vi "[Your Turn] Running Average Using Stacked Shift Register.vi"() -> ()   [LabVIEW 2019]
uses:
  <vilib>/DAQmx/read.llb/DAQmx Read (Analog DBL 1Chan 1Samp).vi
  <vilib>/DAQmx/create/channels.llb/DAQmx Create Channel (AI-Temperature-Thermocouple).vi
  <vilib>/DAQmx/configure/timing.llb/DAQmx Timing (Sample Clock).vi
  <vilib>/DAQmx/miscellaneous.llb/DAQmx Fill In Error Info.vi
panel:
  out "Temperature Chart":dbl(graph)
  out "Average Temperature Chart":dbl(graph)
  in  "Stop":bool
  in  "Thermocouple Channel":tag="PCI-6221/ai0"
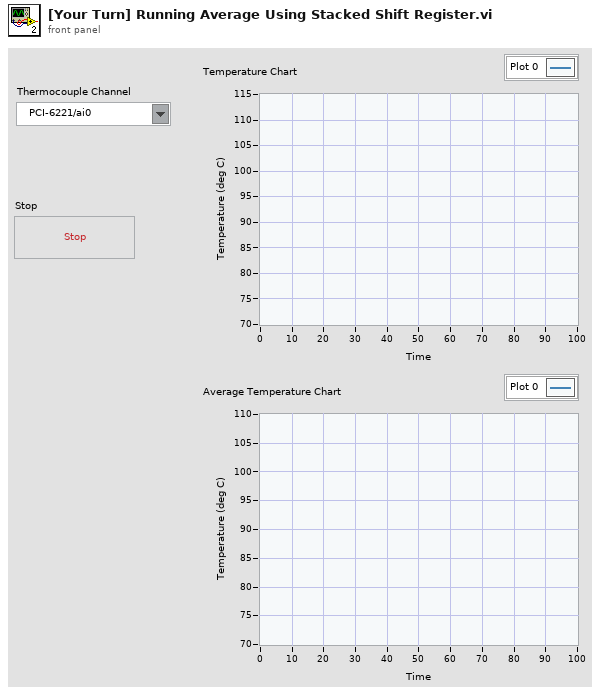
[diagram p1: front panel]
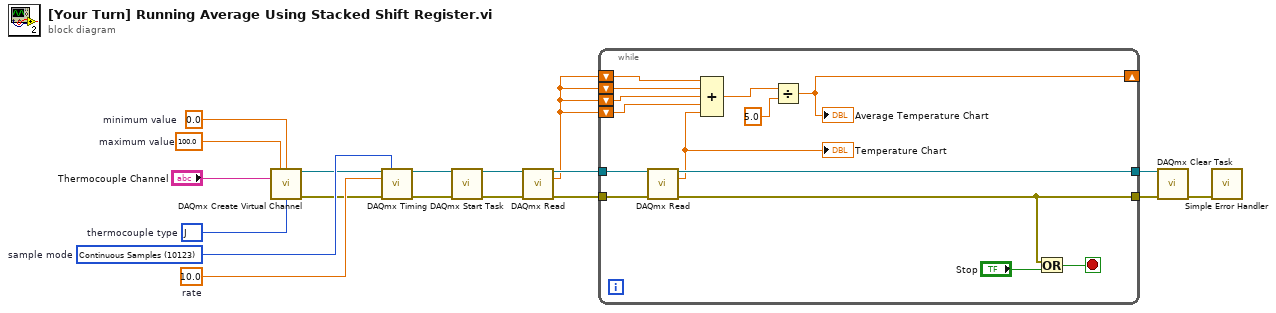
[diagram p0: block diagram]
diagram:
  w7 = 10072 items=["J"=10072, "K"=10073, "N"=10077, "R"=10082, "S"=10085, "T"=10086, "B"=10047, "E"=10055]  # thermocouple type
  w8 = 100.0  # maximum value
  w9 = 0.0  # minimum value
  w17 = 10.0  # rate
  w18 = 10123 items=["Finite Samples"=10178, "Continuous Samples"=10123, "Hardware Timed Single Point"=12522]  # sample mode
  n1 = call-poly <vilib>:"DAQmx Create Virtual Channel.vi"("maximum value"=w8, "minimum value"=w9, "physical channels"="Thermocouple Channel", "thermocouple type"=w7) -> ("task out"=w16:refnum<k21>, "error out"=w15:errorcluster)  [unwired: 10 in]
  n2 = call-poly <vilib>:"DAQmx Timing.vi"("task/channels in"=w16, "sample mode"=w18, "rate"=w17, "error in"=w15) -> ("task out"=w14:refnum<k21>, "error out"=w13:errorcluster)  [unwired: 10 in]
  n3 = call <vilib>:"DAQmx Start Task.vi"("task/channels in"=w14, "error in"=w13) -> ("task out"=w12:refnum<k21>, "error out"=w11:errorcluster)  [unwired: 12 in]
  n4 = call-poly <vilib>:"DAQmx Read.vi"("task/channels in"=w12, "error in"=w11) -> ("task out"=w6:refnum<k21>, "data"=w1:dbl, "error out"=w5:errorcluster)  [unwired: 11 in]
  n5 = while {
    tunnel: w6 -> [w32]
    tunnel: w5 -> [w31]
    shift-right: [w25] -> _
    shift-left: w1 -> [w30]
    shift-left: w1 -> [w29]
    tunnel: [w28] -> w4
    tunnel: [w24] -> w3
    shift-left: w1 -> [w21]
    shift-left: w1 -> [w20]
    stop <- w22 stop-if-true
    n6 = call-poly <vilib>:"DAQmx Read.vi"("task/channels in"=w32, "error in"=w31) -> ("task out"=w28:refnum<k21>, "data"=w19:dbl, "error out"=w24:errorcluster)  [unwired: 11 in]
    "Temperature Chart" <- w19
    n7 = Compound Arithmetic op=ADD(w30, w29, w21, w20, w19) -> (w27:dbl)
    n8 = Divide(x=w27, y=5.0) -> (x/y=w25:dbl)
    "Average Temperature Chart" <- w25
    n9 = Or(x=w24, y="Stop") -> (x .or. y?=w22:bool)
  }
  n10 = call <vilib>:"DAQmx Clear Task.vi"("task in"=w4, "error in"=w3) -> ("error out"=w2:errorcluster)  [unwired: 13 in]
  n11 = call <vilib>:"Simple Error Handler.vi"("error in (no error)"=w2) -> ()  [unwired: 4 in, 5 out]
